vi "Test Launch.vi"() -> ()   [LabVIEW 2019, in "Test.lvlib"]
uses:
  Test.lvlib
  Test/Test.lvclass
  C:/Program Files (x86)/National Instruments/LabVIEW 2019/vi.lib/MGI/Panel Manager/Panel Actor/Panel Actor/Panel Actor.lvclass
  <vilib>/MGI/Panel Manager/Panel/Window Position/Reference Position/Alignment.ctl
  <vilib>/MGI/Panel Manager/Panel/Window Position/Reference Position/Horizontal Alignment.ctl
  <vilib>/MGI/Panel Manager/Panel/Window Position/Reference Position/Vertical Alignment.ctl
  Test Messages/Receive IP Msg/Get Connected IP Msg.lvclass/Get Connected IP Msg.ctl
  <vilib>/ActorFramework/Message Enqueuer/Message Enqueuer.lvclass/Message Enqueuer.ctl
  <vilib>/MGI/Panel Manager/Panel/Window Position/Reference Position/Offset/Absolute Offset/No Offset.vi
  <vilib>/ActorFramework/Message Enqueuer/Enqueue.vi
  <vilib>/MGI/Panel Manager/Panel/Window Position/Reference Position/Offset/Absolute Offset/Absolute Offset.lvclass
  C:/Program Files (x86)/National Instruments/LabVIEW 2019/vi.lib/MGI/Panel Manager/Panel/Window Position/Reference Position/Offset/Offset.lvclass
  <vilib>/MGI/Panel Manager/Panel/Window Position/Reference Position/Ref Display/Ref Display.lvclass
  C:/Program Files (x86)/National Instruments/LabVIEW 2019/vi.lib/MGI/Panel Manager/Panel/Window Position/Window Position.lvclass
  Test Messages/Receive IP Msg/Get Connected IP Msg.lvclass
  C:/Program Files (x86)/National Instruments/LabVIEW 2019/vi.lib/ActorFramework/Message/Message.lvclass
  <vilib>/MGI/Panel Manager/Panel/Window Position/Reference Position/Ref Display/Ref Display.vi
  <vilib>/MGI/Panel Manager/Panel Actor/Panel Actor/Launch Root Panel Window.vi
  <vilib>/ActorFramework/Message Priority Queue/Priority Enqueue.vi
  <vilib>/MGI/Panel Manager/Panel Actor/Panel Actor/Panel Actor.lvclass
  <vilib>/MGI/Panel Manager/Panel/Panel.lvlib
  <vilib>/MGI/Panel Manager/Panel/Window Position/Reference Position/Reference Position.lvclass
  <vilib>/ActorFramework/Stop Msg/Stop Msg.lvclass
  <vilib>/ni/Actors/Network Endpoint Actors/Protocols/Network Stream Strategy/Network Stream Initiator/Network Stream Initiator.lvclass
  C:/Program Files (x86)/National Instruments/LabVIEW 2019/vi.lib/ni/Actors/Network Endpoint Actors/Abstract Classes/Message Stream/Message Stream.lvclass
  C:/Program Files (x86)/National Instruments/LabVIEW 2019/vi.lib/MGI/Panel Manager/Panel/Window Position/Reference Position/Reference Position.lvclass
  C:/Program Files (x86)/National Instruments/LabVIEW 2019/vi.lib/MGI/Monitored Actor/Monitored Actor/Monitored Actor/Monitored Actor.lvclass
  C:/Program Files (x86)/National Instruments/LabVIEW 2019/vi.lib/ActorFramework/Actor/Actor.lvclass
panel:
  in  "Send info":bool
  # "Cobra Test"
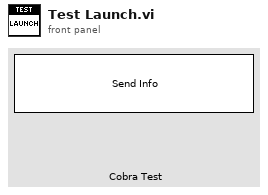
[diagram p1: front panel]
types:
  T1 = enum32{"Invalid", "Standard", "Closed", "Hidden", "Minimized", "Maximized"}
  T2 = typedef "Panel.lvlib/Reference Position.lvclass/Alignment.ctl" = cluster{"Horizontal":T3, "Vertical":T4}
  T3 = typedef "Panel.lvlib/Reference Position.lvclass/Horizontal Alignment.ctl" = enum16{"Left", "Center", "Right"}
  T4 = typedef "Panel.lvlib/Reference Position.lvclass/Vertical Alignment.ctl" = enum16{"Top", "Center", "Bottom"}
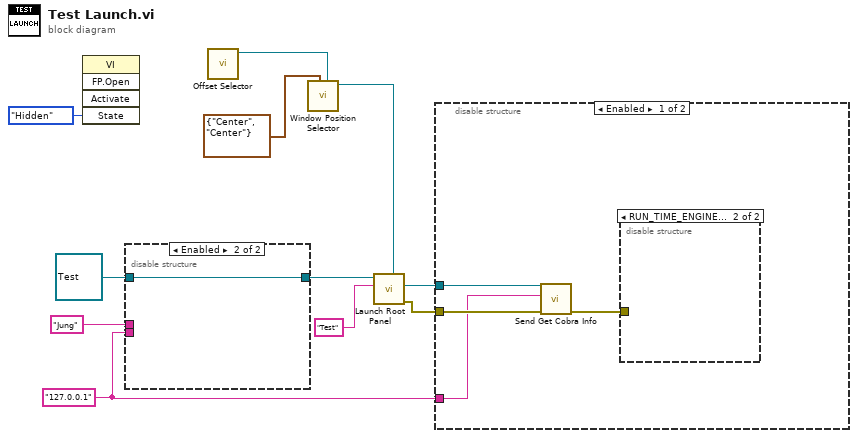
[diagram p0: block diagram]
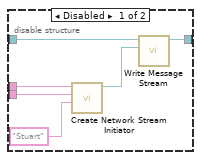
[diagram p2: hidden frame]
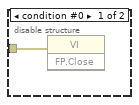
[diagram p3: hidden frame]
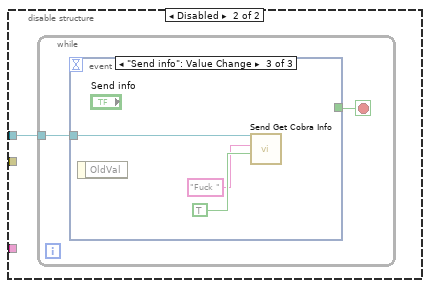
[diagram p4: hidden frame]
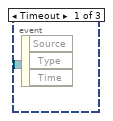
[diagram p5: hidden frame]
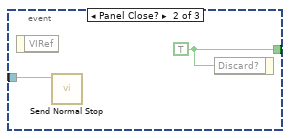
[diagram p6: hidden frame]
diagram:
  w1 = "127.0.0.1" ("IP Address")
  n1 = invoke class="VI" method="FP.Open"("State"=T1."Hidden") -> ()  [unwired: 4 in, 5 out]
  n2 = disable-structure shown="Enabled" {
    disable-tunnel: "Jung" ("Name") -> [w17 _]
    disable-tunnel: refnum<class "Test.lvclass"> refnum ("Test.lvlib:Test.lvclass") -> [w15 w18]
    disable-tunnel: [w14 w18] -> w2
    disable-tunnel: w1 -> [w12 _]
    frame Disabled {
      n3 = call <vilib>:"Create Network Stream Initiator.vi"("Remote Name"="Stuart", "Remote Address"=w12, "Name"=w17) -> ("Network Stream Initiator out"=w13:refnum<class "Network Stream Initiator.lvclass">)  [unwired: 8 in]
      n4 = call "Write Message Stream.vi"("Message Stream"=w13, "Test in"=w15) -> ("Test out"=w14:refnum<class "Test.lvclass">)  [unwired: 9 in]
    }
    frame Enabled {
    }
  }
  n5 = call-poly <vilib>:"Offset Selector.vi"() -> ("Absolute Offset Out"=w11:refnum<class "Absolute Offset.lvclass">)  [unwired: 10 in, 1 out]
  n6 = call-poly <vilib>:"Window Position Selector.vi"("Offset"=w11, "Alignment"=T2 {"Horizontal"=enum."Center", "Vertical"=enum."Center"}) -> ("Ref Display out"=w9:refnum<class "Ref Display.lvclass">)  [unwired: 8 in, 1 out]
  n7 = call-poly <vilib>:"Launch Root Panel.vi"("Window Position (Maximize First Call)"=w9, "Title"="Test", "Panel Actor in"=w2) -> ("Error Out"=w5:errorcluster, "Actor's Enqueuer"=w7:refnum<class "Message Enqueuer.lvclass">)  [unwired: 7 in]
  n8 = disable-structure shown="Enabled" {
    disable-tunnel: w7 -> [w22 w24]
    disable-tunnel: w5 -> [w20 _]
    disable-tunnel: w1 -> [w19 _]
    frame Enabled {
      n9 = call "Send Get Cobra Info.vi"("error in (no error)"=w20, "IP Address"=w19, "Message Enqueuer"=w22) -> ("error out"=w21:errorcluster)  [unwired: 7 in, 1 out]
      n10 = disable-structure shown="RUN_TIME_ENGINE==False" {
        disable-tunnel: w21 -> [w23 _]
        frame condition #0 {
          n11 = invoke class="VI" method="FP.Close"(error in=w23) -> ()  [unwired: 2 in, 3 out]
        }
        frame condition #1 (active) {
        }
      }
    }
    frame Disabled {
      n12 = while {
        tunnel: w24 -> [w25]
        stop <- w26 stop-if-true
        n13 = event shown="[2] \"Send info\": Value Change" {
          selector: _ -> [_ _ _]
          dyn-events: _ -> [_ _ _]
          timeout: _ -> [_ _ _]
          tunnel: [_ w28 _] -> w26
          tunnel: w25 -> [_ w27 w29]
          event Timeout {
            n14 = event-data() -> ()  [unwired: 1 in, 3 out]
          }
          event Panel Close? {
            w28 = TRUE ("Discard?")
            n15 = event-data() -> ()  [unwired: 1 in, 1 out]
            n16 = call <vilib>:"Send Normal Stop.vi"("Message Enqueuer"=w27) -> ()  [unwired: 10 in, 1 out]
            n17 = event-data("Discard?"=w28) -> ()  [unwired: 1 in, 1 out]
          }
          event "Send info": Value Change {
            n18 = event-data() -> ()  [unwired: 1 in, 1 out]
            n19 = call "Send Get Cobra Info.vi"(9:TRUE ("Dual Head"), "IP Address"="Fuck ", "Message Enqueuer"=w29) -> ()  [unwired: 7 in, 2 out]
          }
        }
      }
    }
  }
